vi "Hold Button Motor.vi"(8 "error in (no error)":errorcluster, 9 "Motor Power":dbl, 10 "Boolean":bool=TRUE, 11 "refnum name":string="My Motor RefNum") -> ()   [LabVIEW 2016, in "Huskie Swerve.lvlib"]
uses:
  Huskie Swerve.lvlib
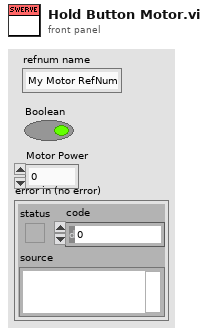
[diagram p1: front panel]
types:
  T1 = typedef "WPI_MotorControlDeviceRef.ctl" = cluster{"DeviceStatus":errorcluster, "Type":T2, "PWM":cluster{"PWM Channel":T3, "DeadBand":T4}, "CAN":cluster{"Device Number":u8, "SetOutput VI Ref":variant, "GetOutput VI Ref":variant, "Enable VI Ref":variant, "Disable VI Ref":variant, "Data":variant}, "Invert":bool}
  T2 = typedef "WPI_MotorControlType.ctl" = enum16{"PWM", "CAN"}
  T3 = typedef "FPGA_DIOPWMChannel.ctl" = enum8{"PWM 0", "PWM 1", "PWM 2", "PWM 3", "PWM 4", "PWM 5", "PWM 6", "PWM 7", "PWM 8", "PWM 9", "PWM MXP 0", "PWM MXP 1", "PWM MXP 2", "PWM MXP 3", "PWM MXP 4", "PWM MXP 5", "PWM MXP 6", "PWM MXP 7", "PWM MXP 8", "PWM MXP 9", "Invalid"}
  T4 = typedef "WPI_PWMDeadband.ctl" = cluster{"Name":string, "maxPositivePwm":i32, "minPositivePwm":i32, "centerPwm":i32, "maxNegativePwm":i32, "minNegativePwm":i32, "angularRange":u16}
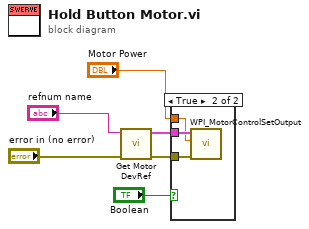
[diagram p0: block diagram]
diagram:
  n1 = call "Get Motor DevRef.vi"("error in (no error)"="error in (no error)", "refnum name"="refnum name") -> ("error out"=w3:errorcluster, "MotorControlDevRef"=w5:T1)  [unwired: 8 in]
  n2 = case shown="True" "Boolean" {
    tunnel: w5 -> [_ w9]
    tunnel: "Motor Power" -> [_ w8]
    tunnel: w3 -> [_ w7]
    frame False {
    }
    frame True {
      n3 = call <vilib>:"WPI_MotorControlSetOutput.vi"("error in (no error)"=w7, "Output"=w8, "MotorControlDevRef"=w9) -> ()  [unwired: 6 in, 3 out]
    }
  }
